vi "BuildTargetBuildSpecification.vi"(8 "error in (no error)":errorcluster, 9 "Name of target (My Computer)":string="My Computer", 10 "Name of build specification (if empty: build all)":string, 11 "Path to project":path) -> (0 "error out":errorcluster, 2 "Generated files":path[](array[path]))   [LabVIEW 2020]
uses:
  <vilib>/AppBuilder/AB_API_Simple/Build (path).vi
  <vilib>/AppBuilder/AB_API_Simple/NI_App_Builder_API.lvlib
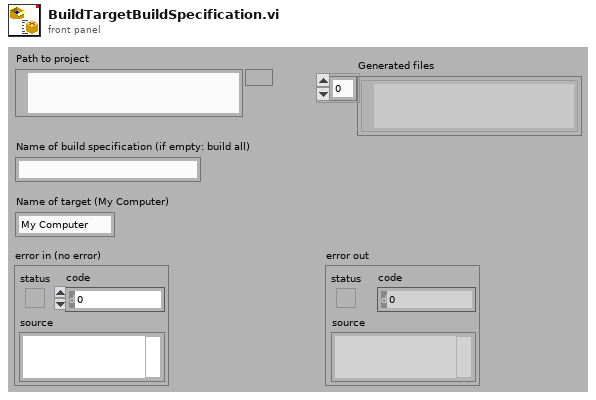
[diagram p1: front panel]
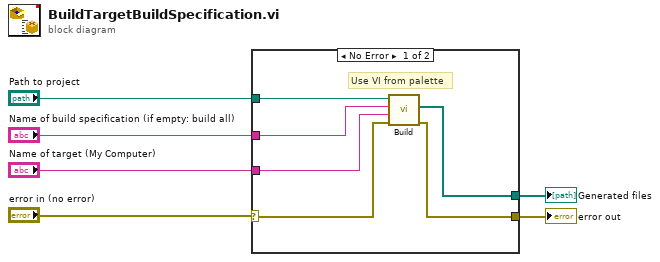
[diagram p0: block diagram]
diagram:
  n1 = case shown="No Error" "error in (no error)" {
    selector: "error in (no error)" -> [w7 w13]
    tunnel: "Path to project" -> [w12 _]
    tunnel: "Name of target (My Computer)" -> [w8 _]
    tunnel: "Name of build specification (if empty: build all)" -> [w9 _]
    tunnel: [w11 _] -> w3
    tunnel: [w10 w13] -> w2
    frame No Error {
      # "Use VI from palette"
      n2 = call-poly <vilib>:"Build.vi"("error in (no error)"=w7, "Name of target (My Computer)"=w8, "Name of build specification (if empty: build all)"=w9, "Path to project"=w12) -> ("error out"=w10:errorcluster, "Generated files"=w11:path[])  [unwired: 6 in]
    }
    frame Error {
    }
  }
  "error out" <- w2
  "Generated files" <- w3
